vi "Example - setup and read wavelength.vi"() -> ()   [LabVIEW 2009, in "HighFinesse WS5.lvlib"]
doc: "Sample program that starts the wavelength meter server, sets a few appopriate options, and then reads the current wavelength until the user hits 'stop'."
uses:
  HighFinesse WS5.lvlib
panel:
  in  "stop":bool
  out "wavelength (air)":dbl
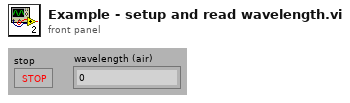
[diagram p1: front panel]
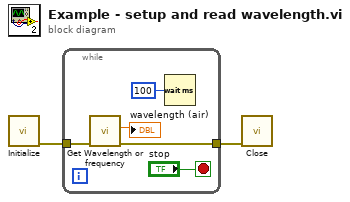
[diagram p0: block diagram]
diagram:
  n1 = call "Initialize.vi"() -> ("error out"=w2:errorcluster)  [unwired: 1 in, 10 out]
  n2 = while {
    tunnel: w2 -> [w7]
    tunnel: [w3] -> w1
    stop <- "stop" stop-if-true
    n3 = call "Get Wavelength or frequency.vi"("error in (no error)"=w7) -> ("error out"=w3:errorcluster, "result"=→"wavelength (air)":dbl)  [unwired: 1 in, 8 out]
    n4 = Wait (ms)(milliseconds to wait=u32 100) -> ()  [unwired: 1 out]
  }
  n5 = call "Close.vi"("error in (no error)"=w1) -> ()  [unwired: 11 out]
